vi "Tokenize by search constant.vi"(10 "search constant":string, 11 "Data":string) -> (3 "Array":string[](array[string]))   [LabVIEW 2013]
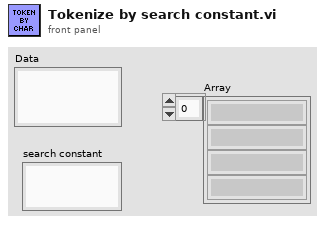
[diagram p1: front panel]
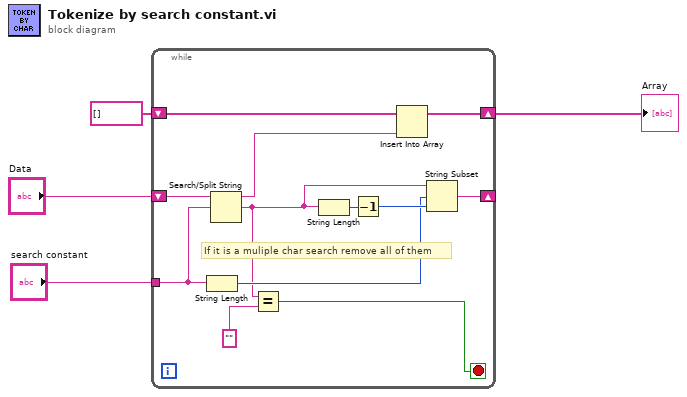
[diagram p0: block diagram]
diagram:
  n1 = while {
    tunnel: "search constant" -> [w7]
    shift-right: [w13] -> _
    shift-left: "Data" -> [w16]
    shift-right: [w15] -> w1
    shift-left: string[] [] -> [w14]
    stop <- w8 stop-if-true
    # "If it is a muliple char search remove all of them"
    n2 = String Length(string=w7) -> (length=w6:i32)
    n3 = Search/Split String(string=w16, search string/char (-)=w7) -> (substring before match=w9:string, match + rest of string=w5:string)  [unwired: 1 in, 1 out]
    n4 = Equal?(x=w5, y="") -> (x = y?=w8:bool)
    n5 = String Length(string=w5) -> (length=w12:i32)
    n6 = Decrement(x=w12) -> (x-1=w11:i32)
    n7 = Insert Into Array(array=w14, new element=w9) -> (w15:string[])  [unwired: 1 in]
    n8 = String Subset(string=w5, offset (0)=w6, length (rest)=w11) -> (substring=w13:string)
  }
  "Array" <- w1
